vi "Enter String SRS Logo.vi"(8 "error in":errorcluster, 10 "String control":string, 11 "Message":string) -> (0 "error out":errorcluster, 2 "String Value":string)   [LabVIEW 2018]
panel:
  in  "OK Button":bool
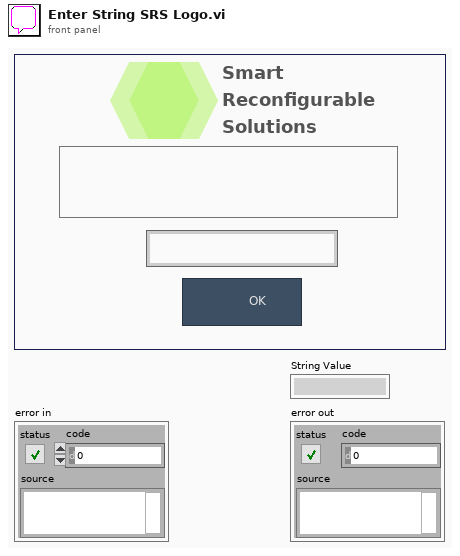
[diagram p1: front panel]
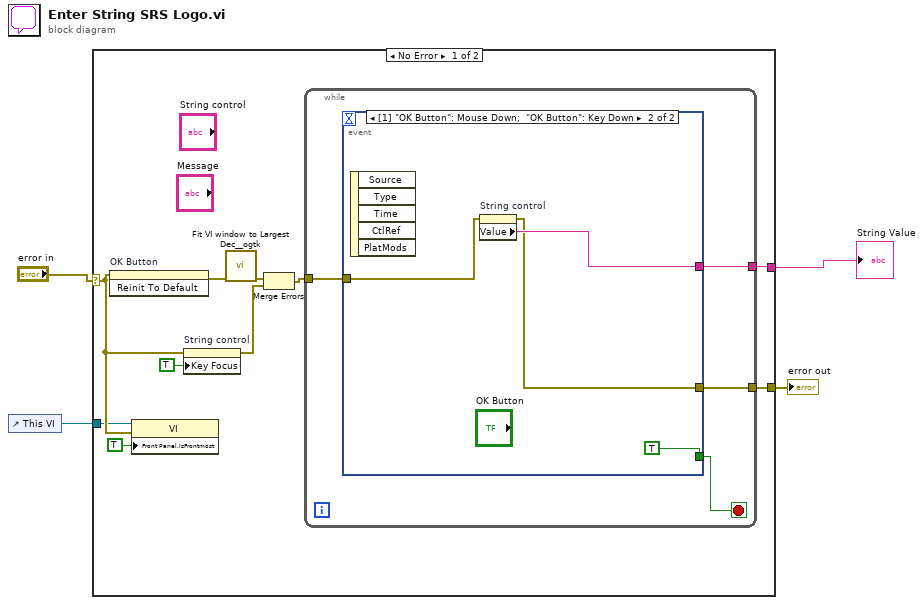
[diagram p0: block diagram]
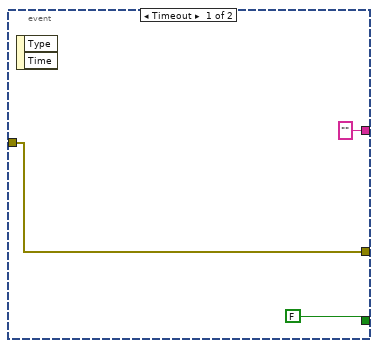
[diagram p2: hidden frame]
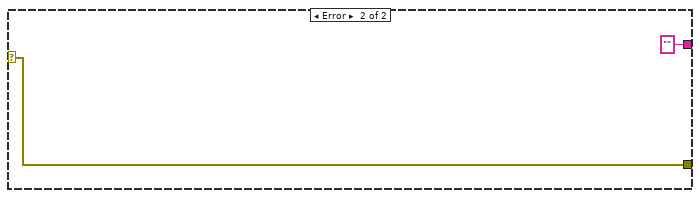
[diagram p3: hidden frame]
diagram:
  n1 = control-ref of="This VI"() -> (w1:refnum<vi>)
  n2 = case shown="No Error" "error in" {
    selector: "error in" -> [w6 w27]
    tunnel: [w13 "" ("Value")] -> w4
    tunnel: [w12 w27] -> w2
    tunnel: w1 -> [w5 _]
    frame No Error {
      n3 = invoke on="OK Button" class="Bool" method="Reinit To Default"(error in=w6) -> (error out=w14:errorcluster)  [unwired: 2 in, 2 out]
      n4 = property class="VI"(reference=w5, error in=w6, "Front Panel.IsFrontmost"=TRUE ("Front Panel Window:Is Frontmost")) -> ()  [unwired: 2 out]
      n5 = property on="String control" class="Str"(error in=w6, "Key Focus"=TRUE) -> (error out=w9:errorcluster)  [unwired: 1 in, 1 out]
      n6 = call <userlib>:"Fit VI window to Largest Dec__ogtk.vi"("error in (no error)"=w14) -> ("error out"=w10:errorcluster)  [unwired: 5 in, 1 out]
      n7 = Merge Errors(w10, w9) -> (w8:errorcluster)
      n8 = while {
        tunnel: w8 -> [w18]
        tunnel: [w17] -> w13
        tunnel: [w16] -> w12
        stop <- w15 stop-if-true
        n9 = event shown="[1] \"OK Button\": Mouse Down;  \"OK Button\": Key Down" {
          selector: _ -> [_ _]
          dyn-events: _ -> [_ _]
          timeout: _ -> [_ _]
          tunnel: w18 -> [w21 w23]
          tunnel: ["" ("Value") w24] -> w17
          tunnel: [w21 w22] -> w16
          tunnel: [FALSE TRUE] -> w15
          event Timeout {
            n10 = event-data() -> ()  [unwired: 1 in, 2 out]
          }
          event "OK Button": Mouse Down; "OK Button": Key Down {
            n11 = event-data() -> ()  [unwired: 1 in, 5 out]
            n12 = property on="String control" class="Str"(error in=w23) -> (error out=w22:errorcluster, "Value"=w24:string)  [unwired: 1 in, 1 out]
          }
        }
      }
    }
    frame Error {
    }
  }
  "String Value" <- w4
  "error out" <- w2
